vi "Create Tree Shortcut Menu.vi"(9 "Selection type":T1, 11 "Menu in":refnum<k9>) -> (0 "error out":errorcluster)   [LabVIEW 2019, in "Panther Dashboard.lvlib"]
uses:
  Panther Dashboard.lvlib
  Selection Type--enum.ctl
  Panther Dashboard--global.vi
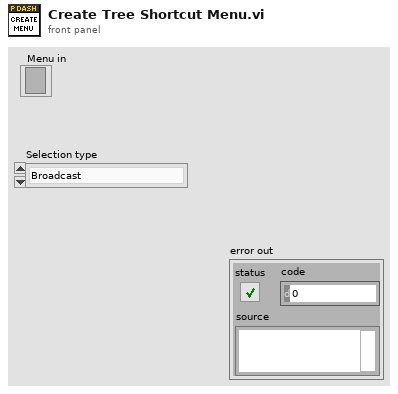
[diagram p1: front panel]
types:
  T1 = typedef "Panther Dashboard.lvlib/Selection Type--enum.ctl" = enum16{"Broadcast", "Request", "Module", "Public API"}
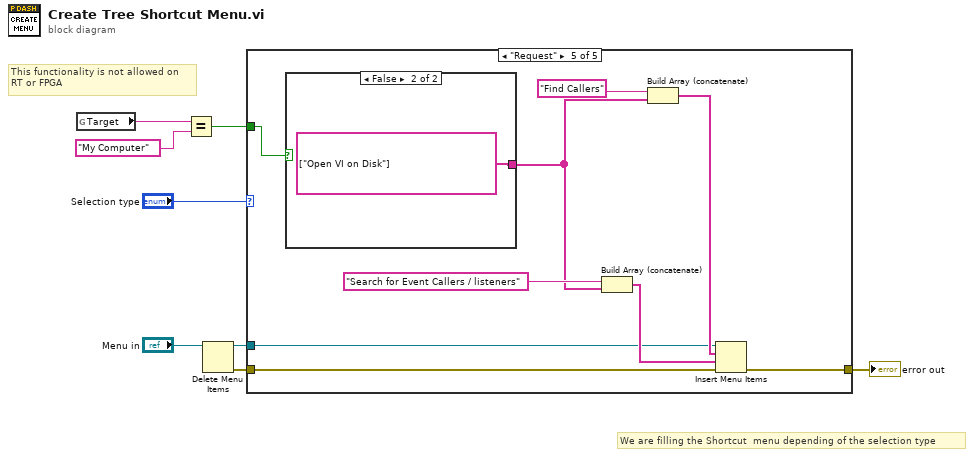
[diagram p0: block diagram]
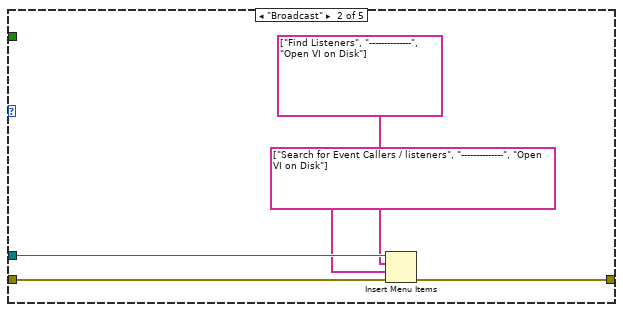
[diagram p3: hidden frame]
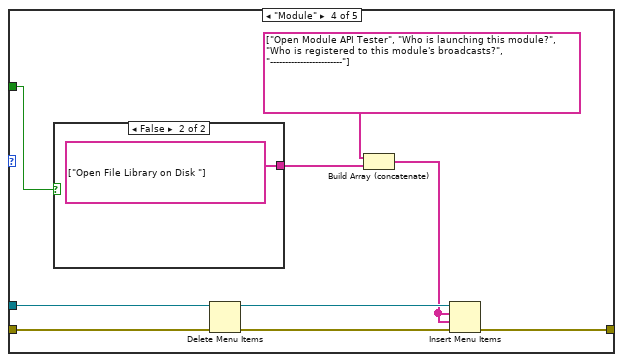
[diagram p5: hidden frame]
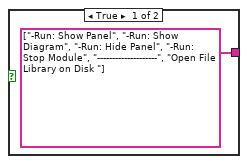
[diagram p6: hidden frame]
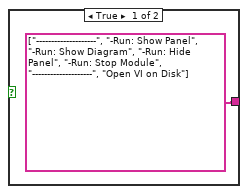
[diagram p7: hidden frame]
diagram:
  # "This functionality is not allowed on\nRT or FPGA"
  # "We are filling the Shortcut  menu depending of the selection type"
  n1 = global read "Panther Dashboard--global.vi" "Target"() -> (w3:string)
  n2 = Equal?(x=w3, y="My Computer") -> (x = y?=w1:bool)
  n3 = Delete Menu Items(9:"Menu in") -> (0:w7:errorcluster, 3:w4:refnum<k9>)  [unwired: 3 in]
  n4 = case shown="\"Request\"" "Selection type" {
    tunnel: [w9 w14 w15 w23 w35] -> w8
    tunnel: w7 -> [w9 w13 w15 w22 w34]
    tunnel: w4 -> [_ w12 _ w17 w29]
    tunnel: w1 -> [_ _ _ w16 w27]
    frame Default {
    }
    frame "Broadcast" {
      n5 = Insert Menu Items(6:w13, 7:string[] ["Search for Event Callers / listeners", "--------------", "Open VI on Disk"], 8:string[] ["Find Listeners", "--------------", "Open VI on Disk"], 9:w12) -> (0:w14:errorcluster)  [unwired: 2 in, 2 out]
    }
    frame "Public API" {
    }
    frame "Module" {
      n6 = case shown="False" w16 {
        tunnel: [string[] ["-Run: Show Panel", "-Run: Show Diagram", "-Run: Hide Panel", "-Run: Stop Module", "--------------------", "Open File Library on Disk "] ("item names") string[] ["Open File Library on Disk "] ("item names")] -> w19
        frame True {
        }
        frame False {
        }
      }
      n7 = Delete Menu Items(6:w22, 9:w17) -> (0:w24:errorcluster, 3:w21:refnum<k9>)  [unwired: 2 in]
      n8 = Build Array (concatenate)(string[] ["Open Module API Tester", "Who is launching this module?", "Who is registered to this module's broadcasts?", "------------------------"] ("item names"), w19) -> (w18:string[])
      n9 = Insert Menu Items(6:w24, 7:w18, 8:w18, 9:w21) -> (0:w23:errorcluster)  [unwired: 2 in, 2 out]
    }
    frame "Request" {
      n10 = case shown="False" w27 {
        tunnel: [string[] ["--------------------", "-Run: Show Panel", "-Run: Show Diagram", "-Run: Hide Panel", "-Run: Stop Module", "--------------------", "Open VI on Disk"] ("item names") string[] ["Open VI on Disk"] ("item names")] -> w28
        frame True {
        }
        frame False {
        }
      }
      n11 = Build Array (concatenate)("Search for Event Callers / listeners", w28) -> (w32:string[])
      n12 = Build Array (concatenate)("Find Callers", w28) -> (w31:string[])
      n13 = Insert Menu Items(6:w34, 7:w32, 8:w31, 9:w29) -> (0:w35:errorcluster)  [unwired: 2 in, 2 out]
    }
  }
  "error out" <- w8
